vi "tm420_sequence_cannula.vi"(0 "Orca Crop":T1={"Horizontal Offset"=0, "Vertical Offset"=0, "Horizontal Width"=1024, "Vertical Width"=1024}, 1 "Orca Exposure":dbl=0.5, 2 "Quit":bool) -> (3 "Image":u16[][](graph))   [LabVIEW 2016]
panel:
  out "Timestamp":dbl
  out "DCAM Version":string
  out "Library Version":string
  out "Frames Per Second":dbl
  out "Error Out":errorcluster {"code" format="%.0x"}
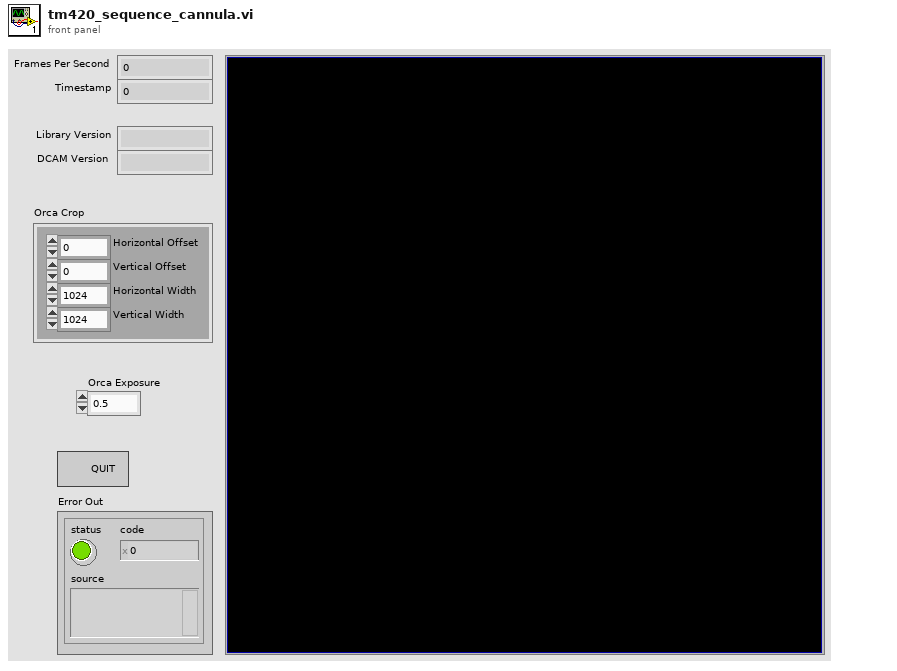
[diagram p1: front panel]
types:
  T1 = cluster{"Horizontal Offset":i32, "Vertical Offset":i32, "Horizontal Width":i32, "Vertical Width":i32}
  T2 = cluster{"Capture Library":string, "DCAM-API":string}
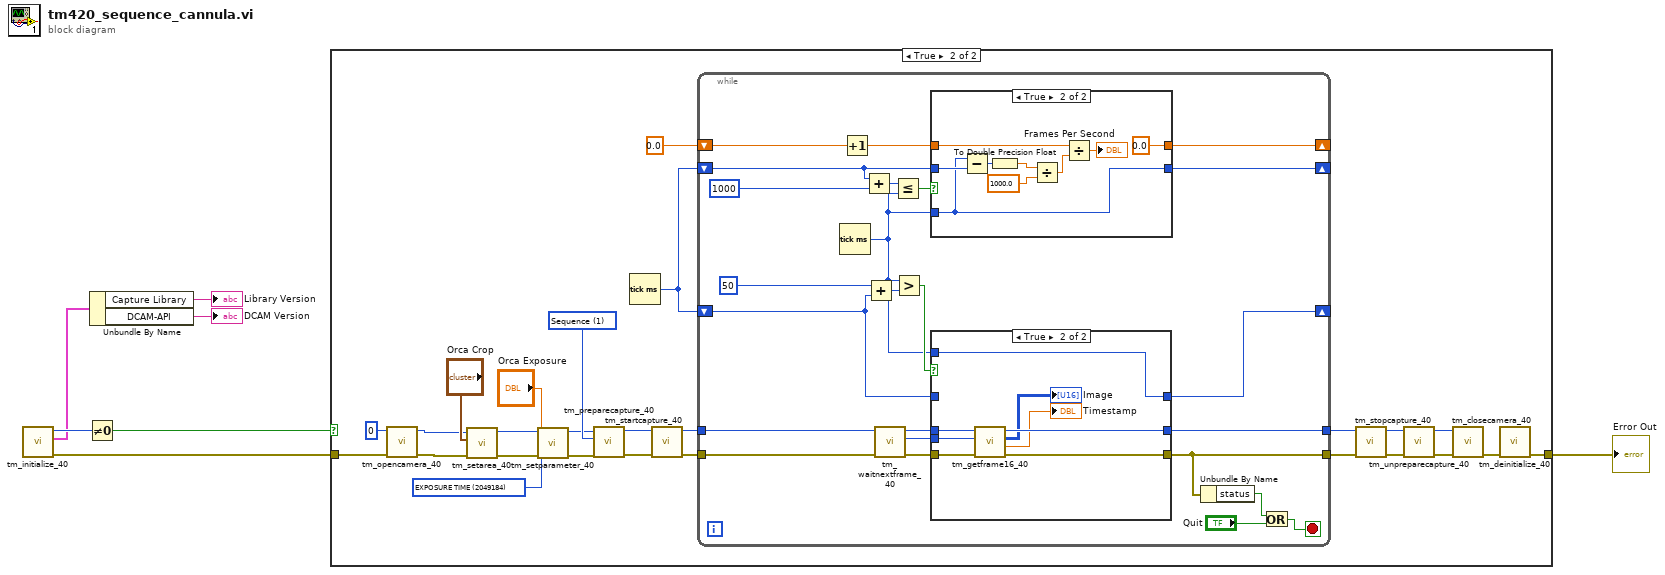
[diagram p0: block diagram]
diagram:
  n1 = call <userlib>:"tm_initialize_40.vi"() -> ("error out"=w5:errorcluster, "Version Info"=w4:T2, "Number Of Cameras"=w6:u32)  [unwired: 8 in, 1 out]
  n2 = Not Equal To 0?(x=w6) -> (x != 0?=w7:bool)
  n3 = Unbundle By Name(w4) -> ("Capture Library"=→"Library Version":string, "DCAM-API"=→"DCAM Version":string)
  n4 = case shown="True" w7 {
    tunnel: w5 -> [w8 w34]
    tunnel: [w8 w18] -> w1
    frame False {
    }
    frame True {
      w14 = u32 2049184 items=["SENSOR MODE"=4212128, "READOUT SPEED"=4211872, "READOUT DIRECTION"=4211904, "TRIGGER GLOBAL EXPOSURE"=2049680, "TRIGGER DELAY"=1066480, "INTERNAL TRIGGER HANDLING"=1066496, "SYNC READOUT SYSTEM BLANK"=1066528, "SENSOR TEMPERATURE"=2115232, "SENSOR COOLER STATUS"=2115280, "EXPOSURE TIME"=2049184, "DEFECT CORRECT MODE"=4670368, "BINNING"=4215968, "INTERNAL LINE SPEED"=4226000, "INTERNAL LINE INTERVAL"=4226016, "NUMBER OF OUTPUT TRIGGER CONNECTOR"=1852320, "OUTPUT TRIGGER SOURCE[0]"=1852576, "OUTPUT TRIGGER SOURCE[1]"=1852832, "OUTPUT TRIGGER SOURCE[2]"=1853088, "OUTPUT TRIGGER POLARITY[0]"=1852592, "OUTPUT TRIGGER POLARITY[1]"=1852848, "OUTPUT TRIGGER POLARITY[2]"=1853104, "OUTPUT TRIGGER ACTIVE[0]"=1852608, "OUTPUT TRIGGER ACTIVE[1]"=1852864, "OUTPUT TRIGGER ACTIVE[2]"=1853120, "OUTPUT TRIGGER DELAY[0]"=1852624, "OUTPUT TRIGGER DELAY[1]"=1852880, "OUTPUT TRIGGER DELAY[2]"=1853136, "OUTPUT TRIGGER PERIOD[0]"=1852640, "OUTPUT TRIGGER PERIOD[1]"=1852896, "OUTPUT TRIGGER PERIOD[2]"=1853152, "OUTPUT TRIGGER KIND[0]"=1852656, "OUTPUT TRIGGER KIND[1]"=1852912, "OUTPUT TRIGGER KIND[2]"=1853168, "OUTPUT TRIGGER BASE SENSOR[0]"=1852672, "OUTPUT TRIGGER BASE SENSOR[1]"=1852928, "OUTPUT TRIGGER BASE SENSOR[2]"=1853184, "OUTPUT TRIGGER PRE HSYNC COUNT"=1852704] ("Parameter")
      w24 = 1 items=["Snap", "Sequence"] ("Capture mode")
      n5 = call <userlib>:"tm_opencamera_40.vi"("error in (no error)"=w34, "Camera Index"=u32 0) -> ("error out"=w11:errorcluster, "Handle out"=w12:u32)  [unwired: 7 in, 1 out]
      n6 = call <userlib>:"tm_setarea_40.vi"("error in (no error)"=w11, "Sub Region"="Orca Crop", "Handle in"=w12) -> ("error out"=w15:errorcluster, "Handle out"=w16:u32)  [unwired: 7 in]
      n7 = call <userlib>:"tm_setparameter_40.vi"("error in (no error)"=w15, "Value in"="Orca Exposure", "Parameter"=w14, "Handle in"=w16) -> ("error out"=w9:errorcluster, "Handle out"=w10:u32)  [unwired: 6 in]
      n8 = call <userlib>:"tm_preparecapture_40.vi"("error in (no error)"=w9, "Capture mode"=w24, "Handle in"=w10) -> ("error out"=w22:errorcluster, "Handle out"=w23:u32)  [unwired: 5 in, 2 out]
      n9 = Tick Count (ms)() -> (millisecond timer value=w20:u32)
      n10 = call <userlib>:"tm_startcapture_40.vi"("error in (no error)"=w22, "Handle in"=w23) -> ("error out"=w25:errorcluster, "Handle out"=w26:u32)  [unwired: 8 in]
      n11 = while {
        tunnel: [w39] -> w29
        tunnel: [w40] -> w30
        tunnel: w26 -> [w36]
        tunnel: w25 -> [w35]
        shift-right: [w55] -> _
        shift-left: w20 -> [w52]
        shift-right: [w56] -> _
        shift-left: 0.0 -> [w49]
        shift-right: [w38] -> _
        shift-left: w20 -> [w41]
        stop <- w37 stop-if-true
        n12 = Tick Count (ms)() -> (millisecond timer value=w42:u32)
        n13 = Increment(x=w49) -> (x+1=w50:dbl)
        n14 = Add(x=w52, y=u32 1000) -> (x+y=w54:u32)
        n15 = Add(x=u32 50, y=w41) -> (x+y=w44:u32)
        n16 = call <userlib>:"tm_waitnextframe_40.vi"("error in (no error)"=w35, "Handle in"=w36) -> ("error out"=w47:errorcluster, "Frame Index"=w46:i32, "Handle out"=w48:u32)  [unwired: 6 in, 1 out]
        n17 = Less Or Equal?(x=w54, y=w42) -> (x <= y?=w51:bool)
        n18 = Greater?(x=w42, y=w44) -> (0:w43:bool)
        n19 = case shown="True" w51 {
          tunnel: w52 -> [w71 w74]
          tunnel: [w71 w72] -> w55
          tunnel: w50 -> [w70 w78]
          tunnel: w42 -> [_ w72]
          tunnel: [w70 0.0] -> w56
          frame False {
          }
          frame True {
            n20 = Subtract(x=w72, y=w74) -> (x-y=w73:u32)
            n21 = To Double Precision Float(number=w73) -> (double precision float=w80:dbl)
            n22 = Divide(x=w80, y=1000.0) -> (x/y=w77:dbl)
            n23 = Divide(x=w78, y=w77) -> (x/y=→"Frames Per Second":dbl)
          }
        }
        n24 = case shown="True" w43 {
          tunnel: w48 -> [w61 w69]
          tunnel: w47 -> [w60 w68]
          tunnel: w46 -> [_ w62]
          tunnel: w41 -> [w59 _]
          tunnel: w42 -> [_ w67]
          tunnel: [w61 w65] -> w39
          tunnel: [w60 w66] -> w40
          tunnel: [w59 w67] -> w38
          frame False {
          }
          frame True {
            n25 = call <userlib>:"tm_getframe16_40.vi"("error in (no error)"=w68, "Frame Index"=w62, "Handle in"=w69) -> ("error out"=w66:errorcluster, "Timestamp"=→"Timestamp":dbl, "Data"=→"Image":u16[][], "Handle out"=w65:u32)  [unwired: 5 in]
          }
        }
        n26 = Unbundle By Name(w40) -> ("status"=w58:bool)
        n27 = Or(x=w58, y="Quit") -> (x .or. y?=w37:bool)
      }
      n28 = call <userlib>:"tm_stopcapture_40.vi"("error in (no error)"=w30, "Handle in"=w29) -> ("error out"=w27:errorcluster, "Handle out"=w28:u32)  [unwired: 8 in]
      n29 = call <userlib>:"tm_unpreparecapture_40.vi"("error in (no error)"=w27, "Handle in"=w28) -> ("error out"=w32:errorcluster, "Handle out"=w31:u32)  [unwired: 8 in]
      n30 = call <userlib>:"tm_closecamera_40.vi"("error in (no error)"=w32, "Handle in"=w31) -> ("error out"=w19:errorcluster)  [unwired: 9 in]
      n31 = call <userlib>:"tm_deinitialize_40.vi"("error in (no error)"=w19) -> ("error out"=w18:errorcluster)  [unwired: 10 in]
    }
  }
  "Error Out" <- w1
